vi "initialize target with engines.vi"(8 "error in (no error)":errorcluster, 9 "timeout in ms (-1)":i32, 10 "engines":T1[](array[typedef]), 11 "PL_Target Configuration in":refnum<class "PL_Target Configuration.lvclass">) -> (0 "error out":errorcluster, 2 "Array":refnum<class "Engine Runtime Interface.lvclass">[](array[class]), 3 "PL_Target Runtime out":refnum<class "PL_Target Runtime.lvclass">)   [LabVIEW 2014, in "PL_Target Runtime.lvclass"]
uses:
  PL_Target Runtime.lvclass
  target configuration/PL_Target Configuration.lvclass
  platypus configuration/engines cluster.ctl
  <vilib>/NI/Module Execution Interface/Engine Configuration/engine configuration.lvclass
  <vilib>/NI/Tag Bus Module Framework/module configuration/TBM module configuration.lvclass
  <vilib>/NI/Module Execution Interface/Engine Runtime/Engine Runtime Interface.lvclass
  platypus configuration/PLConfigurationSerializer.lvlib
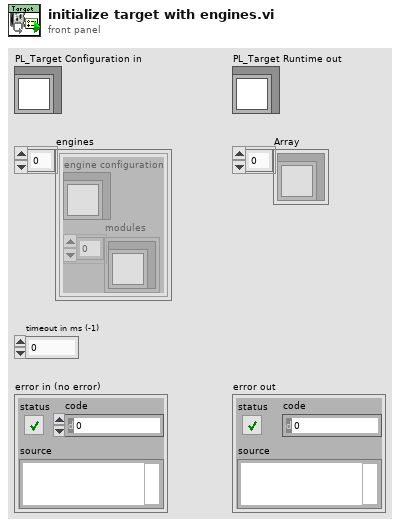
[diagram p1: front panel]
types:
  T1 = typedef "PLConfigurationSerializer.lvlib/engines cluster.ctl" = cluster{"engine configuration":refnum<class "engine configuration.lvclass">, "modules":refnum<class "TBM module configuration.lvclass">[]}
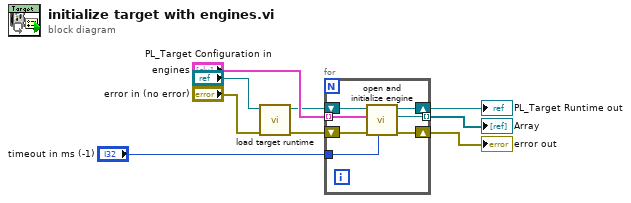
[diagram p0: block diagram]
diagram:
  n1 = call "load target runtime.vi"("error in"="error in (no error)", "target configuration"="PL_Target Configuration in") -> ("error out"=w7:errorcluster, "target runtime"=w1:refnum<class "PL_Target Runtime.lvclass">)  [unwired: 8 in]
  n2 = for {
    tunnel: "engines" -> [w16] mode=indexing
    shift-right: [w12] -> w5
    shift-left: w7 -> [w14]
    tunnel: "timeout in ms (-1)" -> [w13]
    tunnel: [w11] -> w4 mode=indexing
    shift-right: [w10] -> w3
    shift-left: w1 -> [w15]
    n3 = call "open and initialize engine.vi"("timeout in ms"=w13, "error in"=w14, "engine configuration in"=w16, "Target Runtime in"=w15) -> ("error out"=w12:errorcluster, "Engine Runtime Interface out"=w11:refnum<class "Engine Runtime Interface.lvclass">, "Target Runtime out"=w10:refnum<class "PL_Target Runtime.lvclass">)  [unwired: 5 in]
  }
  "error out" <- w5
  "Array" <- w4
  "PL_Target Runtime out" <- w3
